vi "TEST - Boolean Trigger.vi"(8 "error in (no error)":errorcluster) -> (0 "error out":errorcluster, 2 "passed":bool)   [LabVIEW 2020, in "test_openg_boolean.lvlib"]
uses:
  <vilib>/addons/_JKI Toolkits/Caraya/classes/Assert/Assert True.vi
  test_openg_boolean.lvlib
  <vilib>/addons/_JKI Toolkits/Caraya/classes/Test/Test.lvclass
  <vilib>/addons/_JKI Toolkits/Caraya/classes/Assert/Assert.lvclass
  source/library/openg_boolean.lvlib
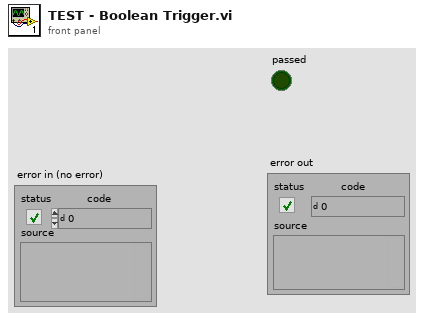
[diagram p1: front panel]
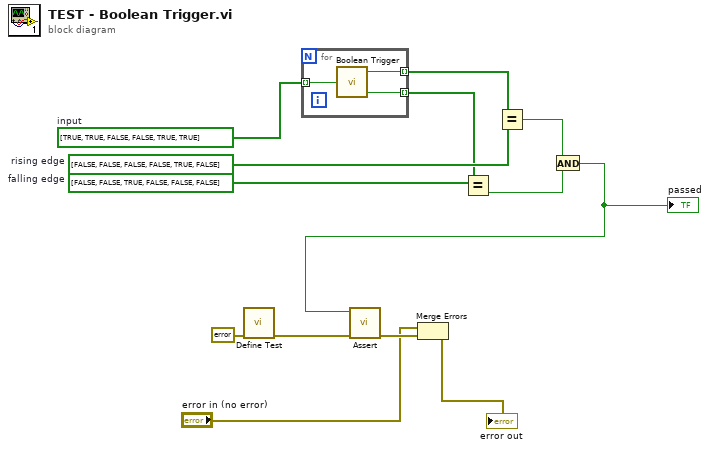
[diagram p0: block diagram]
diagram:
  w6 = bool[] [FALSE, FALSE, TRUE, FALSE, FALSE, FALSE]  # falling edge
  w8 = bool[] [FALSE, FALSE, FALSE, FALSE, TRUE, FALSE]  # rising edge
  w10 = bool[] [TRUE, TRUE, FALSE, FALSE, TRUE, TRUE]  # input
  n1 = call <vilib>:"Define Test.vi"("error in (no error)"=errorcluster {"status"=FALSE, "code"=0, "source"=""}) -> ("error out"=w12:errorcluster)  [unwired: 9 in, 1 out]
  n2 = for {
    tunnel: w10 -> [w16] mode=indexing
    tunnel: [w15] -> w9 mode=indexing
    tunnel: [w14] -> w7 mode=indexing
    n3 = call "Boolean Trigger.vi"("Boolean Input"=w16) -> ("Rising Edge"=w15:bool, "Falling Edge"=w14:bool)  [unwired: 1 in]
  }
  n4 = Equal?(x=w7, y=w6) -> (x = y?=w4:bool)
  n5 = Equal?(x=w9, y=w8) -> (x = y?=w5:bool)
  n6 = And(x=w5, y=w4) -> (x .and. y?=w3:bool)
  "passed" <- w3
  n7 = call-poly <vilib>:"Assert.vi"("error in (no error)"=w12, "True?"=w3) -> ("error out"=w13:errorcluster)  [unwired: 8 in, 1 out]
  n8 = Merge Errors("error in (no error)", w13) -> (→"error out":errorcluster)
